vi "test variant to json.vi"(8 "error in (no error)":errorcluster) -> (0 "error out":errorcluster)   [LabVIEW 2019, in "labview_json_tests.lvlib"]
uses:
  labview_json_tests.lvlib
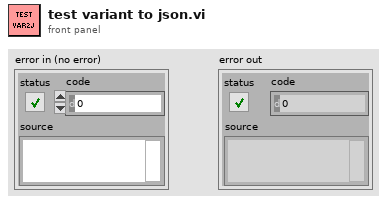
[diagram p1: front panel]
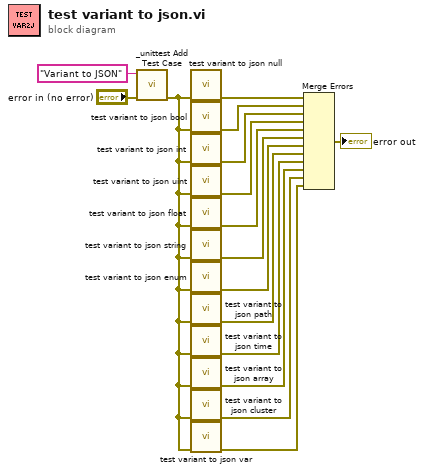
[diagram p0: block diagram]
diagram:
  n1 = call "_unittest Add Test Case.vi"("error in (no error)"="error in (no error)", "Test Case"="Variant to JSON") -> ("error out"=w2:errorcluster)  [unwired: 9 in]
  n2 = call "test variant to json null.vi"("error in (no error)"=w2) -> ("error out"=w8:errorcluster)  [unwired: 10 in]
  n3 = call "test variant to json bool.vi"("error in (no error)"=w2) -> ("error out"=w13:errorcluster)  [unwired: 10 in]
  n4 = call "test variant to json int.vi"("error in (no error)"=w2) -> ("error out"=w12:errorcluster)  [unwired: 10 in]
  n5 = call "test variant to json uint.vi"("error in (no error)"=w2) -> ("error out"=w11:errorcluster)  [unwired: 10 in]
  n6 = call "test variant to json float.vi"("error in (no error)"=w2) -> ("error out"=w10:errorcluster)  [unwired: 10 in]
  n7 = call "test variant to json string.vi"("error in (no error)"=w2) -> ("error out"=w9:errorcluster)  [unwired: 10 in]
  n8 = call "test variant to json enum.vi"("error in (no error)"=w2) -> ("error out"=w3:errorcluster)  [unwired: 10 in]
  n9 = call "test variant to json path.vi"("error in (no error)"=w2) -> ("error out"=w7:errorcluster)  [unwired: 10 in]
  n10 = call "test variant to json time.vi"("error in (no error)"=w2) -> ("error out"=w6:errorcluster)  [unwired: 10 in]
  n11 = call "test variant to json array.vi"("error in (no error)"=w2) -> ("error out"=w5:errorcluster)  [unwired: 10 in]
  n12 = call "test variant to json cluster.vi"("error in (no error)"=w2) -> ("error out"=w4:errorcluster)  [unwired: 10 in]
  n13 = call "test variant to json var.vi"("error in (no error)"=w2) -> ("error out"=w1:errorcluster)  [unwired: 10 in]
  n14 = Merge Errors(w8, w13, w12, w11, w10, w9, w3, w7, w6, w5, w4, w1) -> (→"error out":errorcluster)
